vi "bt-receive_data.vi"(5 "error in (no error)":errorcluster, 9 "data保存":bool) -> (4 "timeout?":bool, 6 "error out":errorcluster, 10 "VISA bytes now":i32)   [LabVIEW 2023, in "bt-interface.lvlib"]
uses:
  bt-interface.lvlib
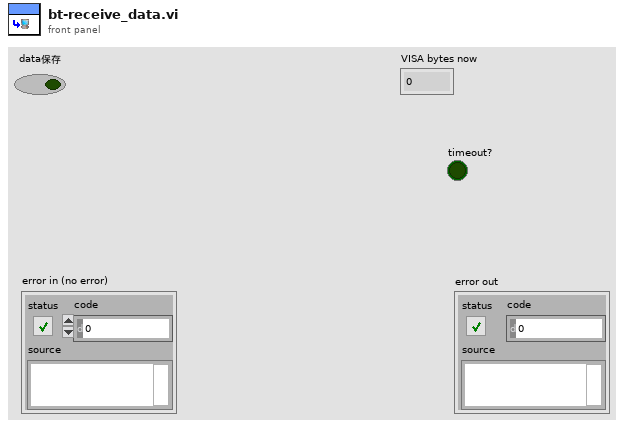
[diagram p1: front panel]
types:
  T1 = enum16{"init", "broadcast_data", "receive_data", "close", "clear_visa"}
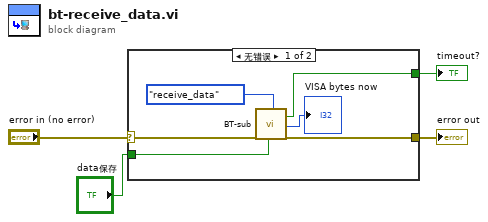
[diagram p0: block diagram]
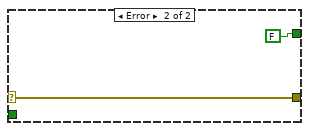
[diagram p2: hidden frame]
diagram:
  n1 = case shown="无错误" "error in (no error)" {
    selector: "error in (no error)" -> [w8 w12]
    tunnel: [w7 w12] -> w3
    tunnel: [w5 FALSE ("timeout?")] -> w2
    tunnel: "data保存" -> [w9 _]
    frame No Error {
      n2 = call "BT-sub.vi"("error in (no error)"=w8, "data存盘"=w9, "mode"=T1."receive_data") -> ("timeout?"=w5:bool, "VISA bytes now"=→"VISA bytes now":i32, "error IO"=w7:errorcluster)  [unwired: 14 in]
    }
    frame Error {
    }
  }
  "error out" <- w3
  "timeout?" <- w2
